vi "Wait.vi"(0 "object in":refnum<class "Application.lvclass">, 2 "Time to wait":dbl=10.0 caption="Time Target (s)", 5 "error in (no error)":errorcluster) -> (14 "object out":refnum<class "Application.lvclass">, 19 "error out":errorcluster)   [LabVIEW 2023, in "Application.lvclass"]
uses:
  Application.lvclass
  Application.lvclass/Application.ctl
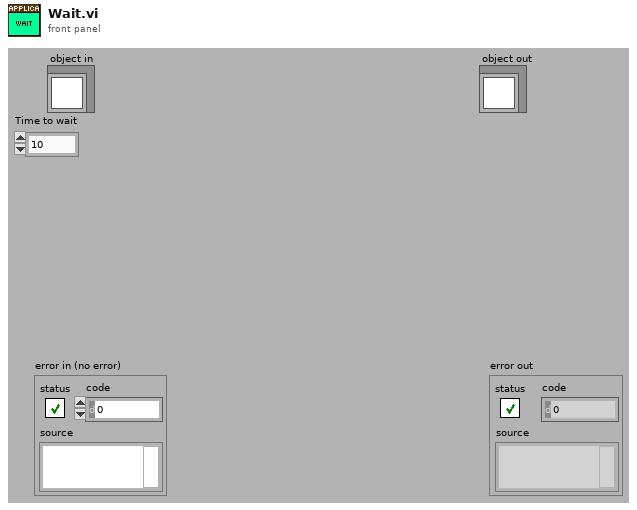
[diagram p1: front panel]
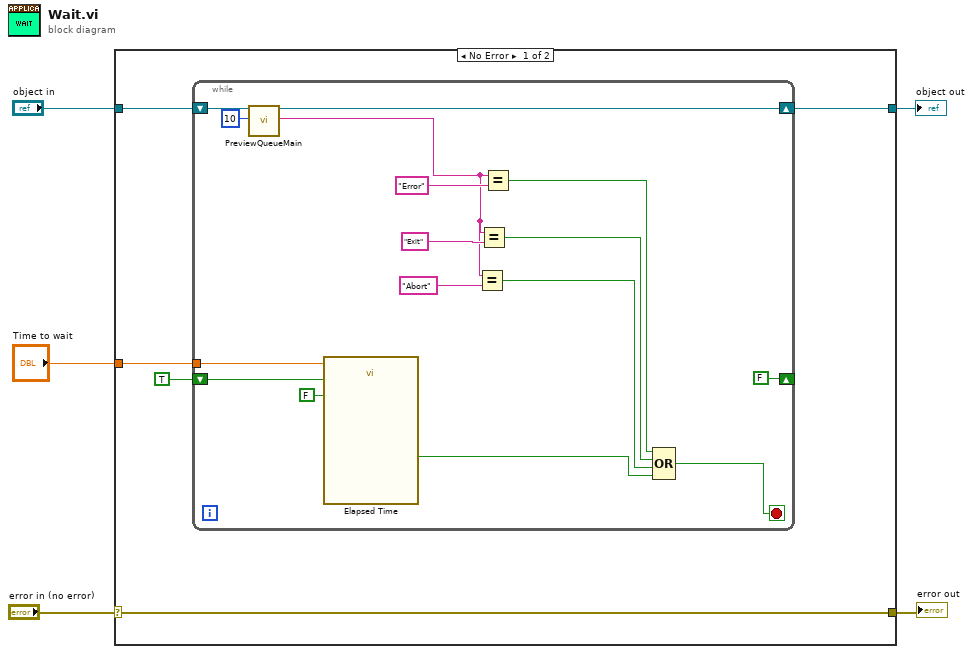
[diagram p0: block diagram]
diagram:
  n1 = case shown="No Error" "error in (no error)" {
    selector: "error in (no error)" -> [w10 w28]
    tunnel: [w10 w28] -> w4
    tunnel: [w9 w27] -> w2
    tunnel: "object in" -> [w8 w27]
    tunnel: "Time to wait" -> [w7 _]
    frame No Error {
      n2 = while {
        shift-right: [w26] -> w9
        shift-left: w8 -> [w25]
        tunnel: w7 -> [w19]
        shift-right: [FALSE ("Reset")] -> _
        shift-left: TRUE ("Reset") -> [w18]
        stop <- w11 stop-if-true
        n3 = call-dynamic "PreviewQueueMain.vi"("object in"=w25, "timeout in ms (-1)"=10) -> ("object out"=w26:refnum<class "Application.lvclass">, "Message"=w21:string)  [unwired: 14 in, 2 out]
        n4 = call "Elapsed Time"("Time Target (s)"=w19, "Reset"=w18, "Auto Reset"=FALSE) -> ("Time has Elapsed"=w12:bool)  [unwired: 9 in, 7 out]
        n5 = Equal?(x=w21, y="Abort") -> (x = y?=w13:bool)
        n6 = Equal?(x=w21, y="Exit") -> (x = y?=w14:bool)
        n7 = Equal?(x=w21, y="Error") -> (x = y?=w15:bool)
        n8 = Compound Arithmetic op=OR(w15, w14, w13, w12) -> (w11:bool)
      }
    }
    frame Error {
    }
  }
  "error out" <- w4
  "object out" <- w2
